vi "Measurement Logic.vi"() -> ()   [LabVIEW 2020, in "NI-SCOPE Acquire Waveform.lvlib"]
uses:
  NI-SCOPE Acquire Waveform.lvlib
  Measurement Configuration.ctl
  <instrlib>/niScope/Controls/niScope vertical coupling.ctl
  <instrlib>/niScope/Controls/niScope trigger slope.ctl
  <instrlib>/niScope/Controls/niScope trigger coupling.ctl
  Measurement Results.ctl
  <vilib>/MeasurementLink/MeasurementLink Measurement Server/Classes/MeasurementContext/MeasurementContext.lvclass
  <vilib>/MeasurementLink/MeasurementLink Measurement Server/Classes/MeasurementContext/Reserve Sessions - NPin.vi
  <vilib>/MeasurementLink/MeasurementLink niScope/Create Sessions - 1Sess.vi
  <vilib>/MeasurementLink/MeasurementLink niScope/Get Connections - 1Pin 1Conn.vi
  <instrlib>/niScope/Configure/Trigger/niScope Configure Trigger Edge.vi
  <instrlib>/niScope/Acquire/niScope Multi Read WDT.vi
  <vilib>/MeasurementLink/MeasurementLink niScope/MeasurementLink niScope.lvlib
  <vilib>/MeasurementLink/MeasurementLink Session Management/Session Reservation/Session Reservation.lvclass
panel:
  out "Measurement Context out":refnum<class "MeasurementContext.lvclass">
  in  "Measurement Context":refnum<class "MeasurementContext.lvclass">
  out "Measurement Results":T1
  in  "Measurement Configuration":T2={"Pin Names"=[], "Vertical Range"=0.0, "Vertical Coupling"=1, "Input Impedance "=0, "Minimum Sample Rate"=0.0, "Minimum Record Length"=0, "Trigger Source"="", "Trigger Level"=0.0, "Trigger Slope"=0, "Timeout"=0.0, "Trigger Coupling"=1} {"Trigger Coupling" items=["AC"=0, "DC"=1, "HF Reject"=3, "LF Reject"=4, "AC Plus HF Reject"=1001]; "Trigger Slope" items=["Positive", "Negative"]; "Vertical Coupling" items=["AC", "DC", "Ground"]}
  out "error out":errorcluster
  in  "error in":errorcluster
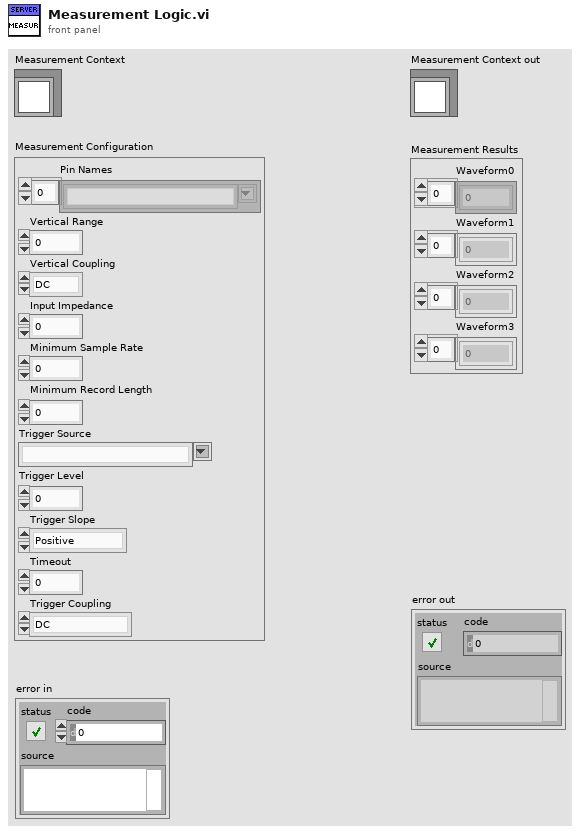
[diagram p1: front panel]
types:
  T1 = typedef "NI-SCOPE Acquire Waveform.lvlib/Measurement Results.ctl" = cluster{"Waveform0":dbl[], "Waveform1":dbl[], "Waveform2":dbl[], "Waveform3":dbl[]}
  T2 = typedef "NI-SCOPE Acquire Waveform.lvlib/Measurement Configuration.ctl" = cluster{"Pin Names":string[], "Vertical Range":dbl, "Vertical Coupling":T3, "Input Impedance ":u32, "Minimum Sample Rate":dbl, "Minimum Record Length":i32, "Trigger Source":string, "Trigger Level":dbl, "Trigger Slope":T4, "Timeout":dbl, "Trigger Coupling":T5}
  T3 = typedef "niScope vertical coupling.ctl" = i32
  T4 = typedef "niScope trigger slope.ctl" = i32
  T5 = typedef "niScope trigger coupling.ctl" = u16
  T6 = typedef "MeasurementLink niScope.lvlib/Connection with Session.ctl" = cluster{"connection":T7, "session":refnum<k15>}
  T7 = typedef "MeasurementLink Session Management.lvlib/Session Reservation.lvclass/Connection.ctl" = cluster{"pin or relay name":string, "site":i32, "instrument type id":string, "channel":string}
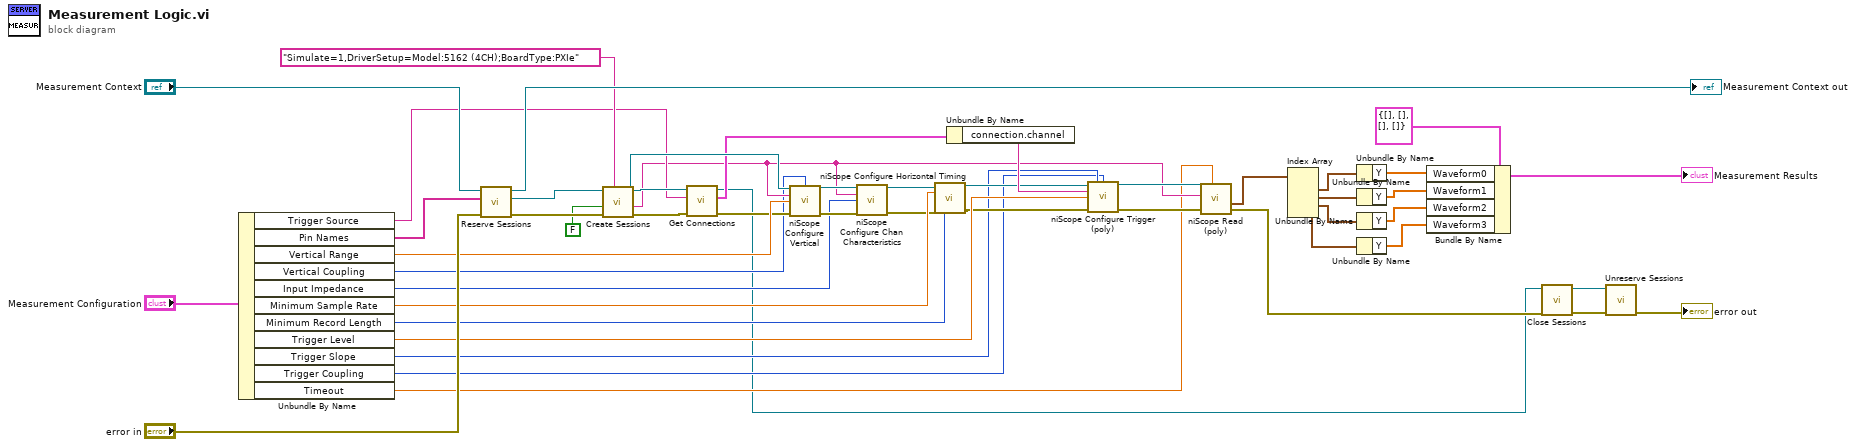
[diagram p0: block diagram]
diagram:
  n1 = Unbundle By Name("Measurement Configuration") -> ("Trigger Source"=w21:string, "Pin Names"=w39:string[], "Vertical Range"=w37:dbl, "Vertical Coupling"=w10:T3, "Input Impedance"=w9:u32, "Minimum Sample Rate"=w35:dbl, "Minimum Record Length"=w32:i32, "Trigger Level"=w27:dbl, "Trigger Slope"=w8:T4, "Trigger Coupling"=w7:T5, "Timeout"=w6:dbl)
  n2 = call-poly <vilib>:"Reserve Sessions.vi"("error in"="error in", "pin or relay names"=w39, "measurement context in"="Measurement Context") -> ("error out"=w43:errorcluster, "session reservation out"=w44:refnum<class "Session Reservation.lvclass">, "measurement context out"=→"Measurement Context out":refnum<class "MeasurementContext.lvclass">)  [unwired: 6 in]
  n3 = call-poly <vilib>:"Create Sessions.vi"("option string"="Simulate=1,DriverSetup=Model:5162 (4CH);BoardType:PXIe", "error in"=w43, "reset"=FALSE, "session reservation in"=w44) -> ("error out"=w24:errorcluster, "channel list"=w11:string, "session"=w38:refnum<k15>, "session reservation out"=w31:refnum<class "Session Reservation.lvclass">)  [unwired: 4 in]
  n4 = call-poly <vilib>:"Get Connections.vi"("error in"=w24, "pin or relay name"=w21, "session reservation in"=w31) -> ("error out"=w23:errorcluster, "connection"=w30:T6, "session reservation out"=w2:refnum<class "Session Reservation.lvclass">)  [unwired: 6 in]
  n5 = call <instrlib>:"niScope Configure Vertical.vi"("instrument handle"=w38, "vertical coupling"=w10, "channels"=w11, "vertical range"=w37, "error in"=w23) -> ("instrument handle out"=w40:refnum<k15>, "error out"=w34:errorcluster)  [unwired: 9 in]
  n6 = call <instrlib>:"niScope Configure Chan Characteristics.vi"("instrument handle"=w40, "channels"=w11, "input impedance"=w9, "error in"=w34) -> ("instrument handle out"=w36:refnum<k15>, "error out"=w33:errorcluster)  [unwired: 10 in]
  n7 = call <instrlib>:"niScope Configure Horizontal Timing.vi"("instrument handle"=w36, "min sample rate"=w35, "error in"=w33, "min record length"=w32) -> ("instrument handle out"=w28:refnum<k15>, "error out"=w22:errorcluster)  [unwired: 10 in]
  n8 = Unbundle By Name(w30) -> ("connection.channel"=w29:string)
  n9 = call-poly <instrlib>:"niScope Configure Trigger (poly).vi"("instrument handle"=w28, "trigger slope"=w8, "trigger coupling"=w7, "trigger source"=w29, "trigger level"=w27, "error in"=w22) -> ("instrument handle out"=w26:refnum<k15>, "error out"=w25:errorcluster)  [unwired: 8 in]
  n10 = call-poly <instrlib>:"niScope Read (poly).vi"("timeout"=w6, "error in"=w25, "channels"=w11, "instrument handle"=w26) -> ("error out"=w3:errorcluster, "wfm"=w20:waveform(dbl)[])  [unwired: 4 in, 2 out]
  n11 = Index Array(array=w20) -> (element #1=w15:waveform(dbl), element #2=w14:waveform(dbl), element #3=w13:waveform(dbl), element #4=w12:waveform(dbl))  [unwired: 4 in]
  n12 = Unbundle By Name(w15) -> ("Y"=w19:dbl[])
  n13 = Unbundle By Name(w14) -> ("Y"=w18:dbl[])
  n14 = Unbundle By Name(w13) -> ("Y"=w17:dbl[])
  n15 = Unbundle By Name(w12) -> ("Y"=w16:dbl[])
  n16 = Bundle By Name(cluster=T1 {"Waveform0"=[], "Waveform1"=[], "Waveform2"=[], "Waveform3"=[]} ("Measurement Results"), "Waveform0"=w19, "Waveform1"=w18, "Waveform2"=w17, "Waveform3"=w16) -> (→"Measurement Results":T1)
  n17 = call <vilib>:"Close Sessions.vi"("error in"=w3, "session reservation in"=w2) -> ("error out"=w4:errorcluster, "session reservation out"=w1:refnum<class "Session Reservation.lvclass">)  [unwired: 8 in]
  n18 = call <vilib>:"Unreserve Sessions.vi"("error in"=w4, "session reservation in"=w1) -> ("error out"=→"error out":errorcluster)  [unwired: 9 in]
